vi "Get Unbundler Output Terminal By Name.vi"(8 "error in (no error)":errorcluster, 10 "Terminal name":string, 11 "Unbundler in":refnum<vi>) -> (0 "error out":errorcluster, 1 "Found?":bool, 2 "Terminal Refnum":refnum<vi>, 3 "Unbundler out":refnum<vi>)   [LabVIEW 2019, in "gRPC Template Creation Utility.lvlib"]
uses:
  gRPC Template Creation Utility.lvlib
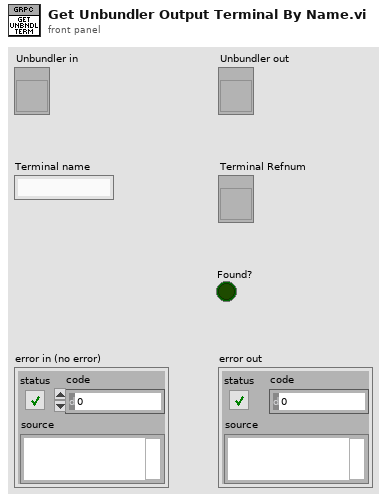
[diagram p1: front panel]
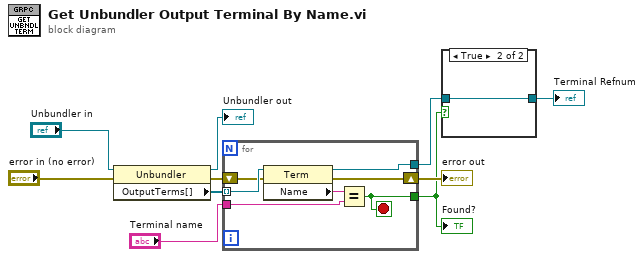
[diagram p0: block diagram]
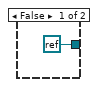
[diagram p2: hidden frame]
diagram:
  n1 = property class="Unbundler"(reference="Unbundler in", error in="error in (no error)") -> (reference out=→"Unbundler out":refnum<vi>, error out=w10:errorcluster, "OutputTerms[]"=w8:refnum<vi>[])
  n2 = for {
    tunnel: w8 -> [w17] mode=indexing
    shift-right: [w15] -> w6
    shift-left: w10 -> [w16]
    tunnel: "Terminal name" -> [w13]
    tunnel: [w12] -> w3
    tunnel: [w11] -> w4
    stop <- w11 stop-if-true
    n3 = property class="Term"(reference=w17, error in=w16) -> (reference out=w12:refnum<vi>, error out=w15:errorcluster, "Name"=w14:string)
    n4 = Equal?(x=w14, y=w13) -> (x = y?=w11:bool)
  }
  "error out" <- w6
  "Found?" <- w4
  n5 = case shown="True" w4 {
    tunnel: w3 -> [_ w19]
    tunnel: [refnum<k0> refnum w19] -> w2
    frame False {
    }
    frame True {
    }
  }
  "Terminal Refnum" <- w2
